vi "Create Bitmap.vi"(8 "error in (no error)":errorcluster caption="错误输入（无错误）", 11 "Screen 输入":refnum<class "Screen.lvclass"> caption="DNL_LabVIEW Object in") -> (0 "error out":errorcluster caption="错误输出", 3 "Screen 输出":refnum<class "Screen.lvclass"> caption="DNL_LabVIEW Object out")   [LabVIEW 2011, in "Screen.lvclass"]
uses:
  Screen.lvclass
  Screen.lvclass/Screen.ctl
  System.Drawing
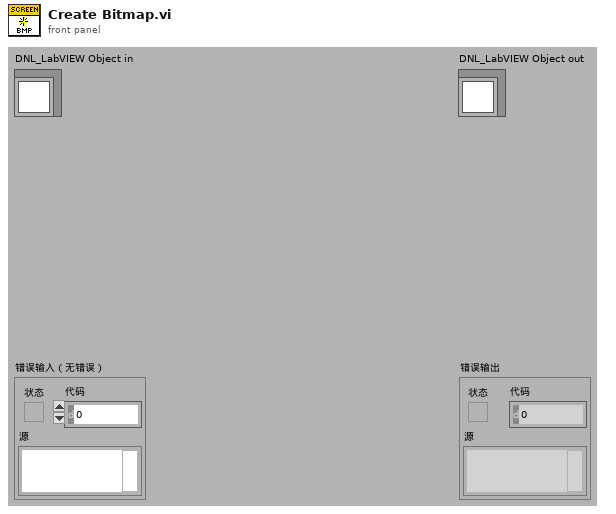
[diagram p1: front panel]
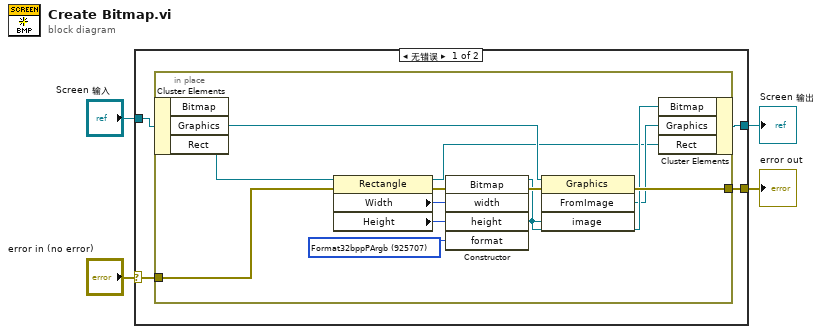
[diagram p0: block diagram]
diagram:
  n1 = case shown="无错误" "error in (no error)" {
    selector: "error in (no error)" -> [w7 w22]
    tunnel: [w6 w22] -> w3
    tunnel: [w5 w21] -> w1
    tunnel: "Screen 输入" -> [w8 w21]
    frame No Error {
      n2 = in-place {
        in-place-border: w7 -> [w10]
        in-place-border: [w20] -> w6
        w15 = 925707 items=["DontCare, Undefined"=0, "Max"=15, "Indexed"=65536, "Gdi"=131072, "Format16bppRgb555"=135173, "Format16bppRgb565"=135174, "Format24bppRgb"=137224, "Format32bppRgb"=139273, "Format1bppIndexed"=196865, "Format4bppIndexed"=197634, "Format8bppIndexed"=198659, "Alpha"=262144, "Format16bppArgb1555"=397319, "PAlpha"=524288, "Format32bppPArgb"=925707, "Extended"=1048576, "Format16bppGrayScale"=1052676, "Format48bppRgb"=1060876, "Format64bppPArgb"=1851406, "Canonical"=2097152, "Format32bppArgb"=2498570, "Format64bppArgb"=3424269] ("format")
        n3 = in-place-cluster #1(w8) -> ("Graphics"=w18:refnum<k24>, "Rect"=w14:refnum<k24>)  [unwired: 1 out]
        n4 = property class="Rectangle"(reference=w14, error in=w10) -> (reference out=w13:refnum<k24>, error out=w9:errorcluster, "Width"=w12:i32, "Height"=w11:i32)
        n5 = constructor class="Bitmap"(error in=w9, "width"=w12, "height"=w11, "format"=w15) -> (reference out=w17:refnum<k24>, error out=w19:errorcluster)  [unwired: 2 in, 4 out]
        n6 = invoke class="Graphics" method="FromImage"(reference=w18, error in=w19, "image"=w17) -> (error out=w20:errorcluster, "FromImage"=w16:refnum<k24>)  [unwired: 1 in, 2 out]
        n7 = in-place-cluster #1("Bitmap"=w17, "Graphics"=w16, "Rect"=w13) -> (w5:refnum<class "Screen.lvclass">)
      }
    }
    frame Error {
    }
  }
  "error out" <- w3
  "Screen 输出" <- w1
